vi "Configure State Trigger.vi"(8 "error in (no error)":errorcluster {"code" format="%.0x"}, 9 "Condition (False)":bool, 10 "Trigger Slope (Positive)":i32(slide), 11 "VISA Resource Name":refnum<visa-resource-name>) -> (0 "error out":errorcluster {"code" format="%.0x"}, 3 "VISA Resource Name Out":refnum<visa-resource-name>)   [LabVIEW 2010, in "Tektronix TDS 3000 Series.lvlib"]
doc: "This VI configures the State trigger. This enables state triggering, which triggers the oscilloscope when the specified condition on one channel (state) is met after a second channel (clock) condition is met.\n\nNotes:\n\n(1) This VI affects instrument behavior only if the Trigger Type is set to State Trigger. Call the Configure Trigger VI to set the Trigger Type before you call this VI."
uses:
  <instrlib>/Tektronix TDS 3000 Series/Tektronix TDS 3000 Series.lvlib
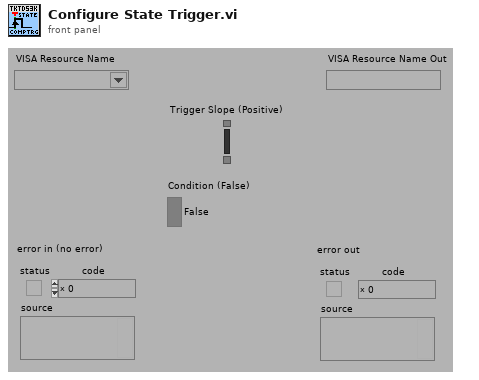
[diagram p1: front panel]
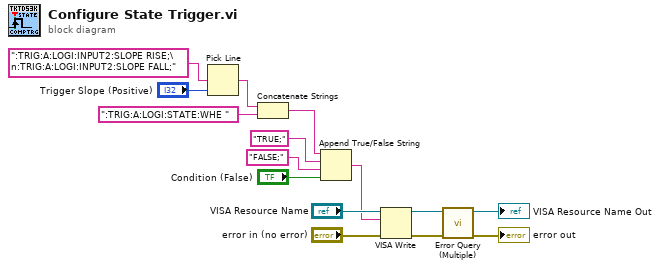
[diagram p0: block diagram]
diagram:
  n1 = Pick Line(multi-line string=":TRIG:A:LOGI:INPUT2:SLOPE RISE;\n:TRIG:A:LOGI:INPUT2:SLOPE FALL;", line index="Trigger Slope (Positive)") -> (output string=w11:string)  [unwired: 1 in]
  n2 = Concatenate Strings(w11, ":TRIG:A:LOGI:STATE:WHE " ("string")) -> (w8:string)
  n3 = Append True/False String(1:"Condition (False)", 2:"FALSE;" ("false string"), 3:"TRUE;" ("true string"), 4:w8) -> (0:w9:string)
  n4 = VISA Write(VISA resource name="VISA Resource Name", write buffer=w9, error in (no error)="error in (no error)") -> (VISA resource name out=w4:refnum<visa-resource-name>, error out=w3:errorcluster)  [unwired: 1 out]
  n5 = call <instrlib>:"Error Query (Multiple).vi"("error in (no error)"=w3, "VISA Resource Name"=w4) -> ("error out"=→"error out":errorcluster, "VISA Resource Name Out"=→"VISA Resource Name Out":refnum<visa-resource-name>)  [unwired: 6 in, 2 out]
